vi "Add CommonVIs to System Explorer.vi"(6 "SE Path Cluster In":T1, 8 "error in":errorcluster) -> (0 "error out":errorcluster, 4 "SE Path Cluster In":T1)   [LabVIEW 2026, in "NIVS_CDEW_MetaDataObj.lvclass"]
uses:
  NIVS_CDEW_MetaDataObj.lvclass
  NIVS_CDEW_MetaDataObj.lvclass/NIVS_CDEW_MetaDataObj.ctl
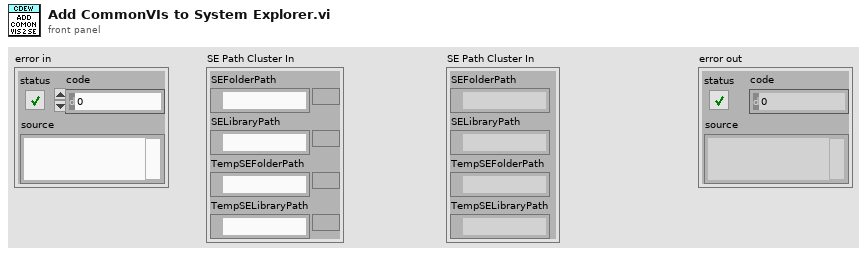
[diagram p1: front panel]
types:
  T1 = cluster{"SEFolderPath":path, "SELibraryPath":path, "TempSEFolderPath":path, "TempSELibraryPath":path}
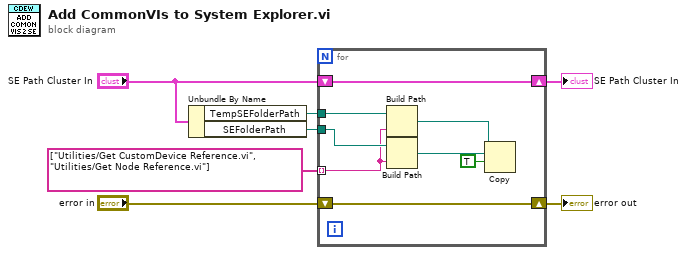
[diagram p0: block diagram]
diagram:
  n1 = Unbundle By Name("SE Path Cluster In") -> ("TempSEFolderPath"=w3:path, "SEFolderPath"=w2:path)
  n2 = for {
    shift-right: [w14] -> w6
    shift-left: "error in" -> [w14]
    shift-right: [w15] -> w7
    shift-left: "SE Path Cluster In" -> [w15]
    tunnel: w2 -> [w13]
    tunnel: w3 -> [w12]
    tunnel: string[] ["Utilities/Get CustomDevice Reference.vi", "Utilities/Get Node Reference.vi"] -> [w9] mode=indexing
    n3 = Build Path(base path=w12, name or relative path=w9) -> (appended path=w11:path)
    n4 = Build Path(base path=w13, name or relative path=w9) -> (appended path=w10:path)
    n5 = Copy(9:TRUE ("overwrite (F)"), 10:w10, 11:w11) -> ()  [unwired: 2 in, 3 out]
  }
  "SE Path Cluster In" <- w7
  "error out" <- w6
